vi "TabControl-EnDis.vi"(8 "Error In":errorcluster, 10 "Page Enabled State":T1(ring), 11 "TabControl in":refnum<vi>) -> (0 "Error Out":errorcluster)   [LabVIEW 2014]
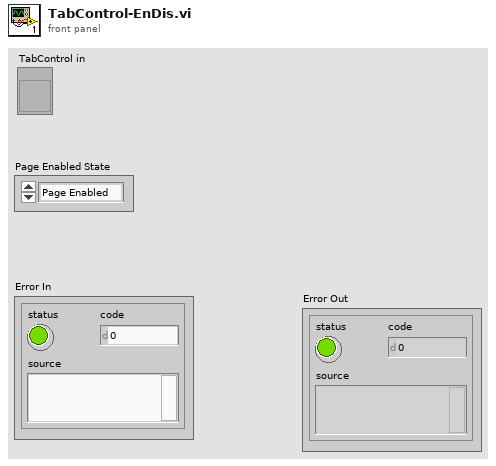
[diagram p1: front panel]
types:
  T1 = enum32{"Page Enabled", "Page Disabled", "Page Disabled & Grayed"}
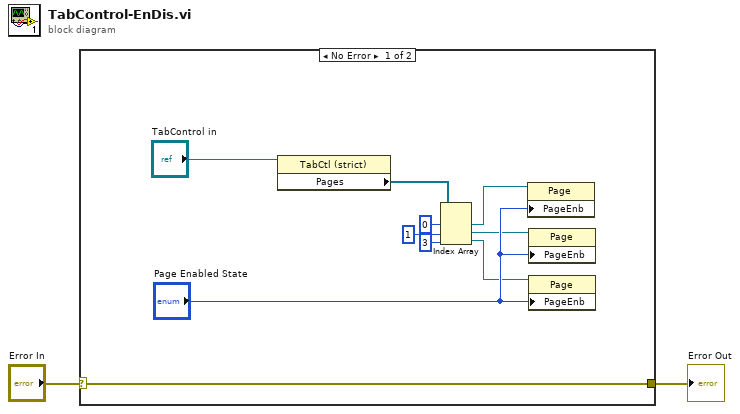
[diagram p0: block diagram]
diagram:
  n1 = case shown="No Error" "Error In" {
    selector: "Error In" -> [w3 w13]
    tunnel: [w3 w13] -> w1
    frame No Error {
      n2 = property on="Property Node" class="TabCtl (strict)"(reference="TabControl in") -> ("Pages"=w5:refnum<vi>[])  [unwired: 1 in, 2 out]
      n3 = Index Array(array=w5, index #1=0 ("index"), index #2=1 ("index"), index #3=3 ("index")) -> (element #1=w9:refnum<vi>, element #2=w10:refnum<vi>, element #3=w11:refnum<vi>)
      n4 = property class="Page"(reference=w9, "PageEnb"="Page Enabled State") -> ()  [unwired: 1 in, 2 out]
      n5 = property class="Page"(reference=w10, "PageEnb"="Page Enabled State") -> ()  [unwired: 1 in, 2 out]
      n6 = property class="Page"(reference=w11, "PageEnb"="Page Enabled State") -> ()  [unwired: 1 in, 2 out]
    }
    frame Error {
    }
  }
  "Error Out" <- w1
